vi "SendAndReceiveTest.vi"(8 "error in (no error)":errorcluster, 11 "SerialPortRef":T1) -> (0 "error out":errorcluster, 1 "Buffer":string, 3 "SerialPortRef 2":T1)   [LabVIEW 2015]
uses:
  <vilib>/Rock Robotics/WPI/SerialPort/WPI_SerialPortRef.ctl
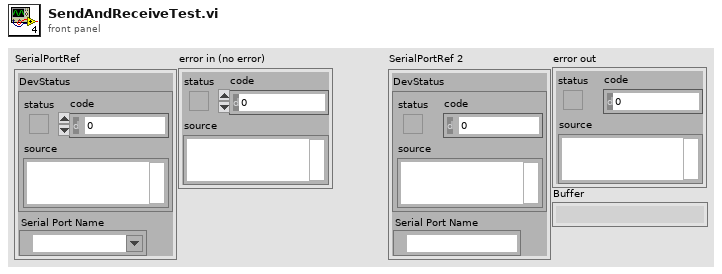
[diagram p1: front panel]
types:
  T1 = typedef "WPI_SerialPortRef.ctl" = cluster{"DevStatus":errorcluster, "Serial Port Name":refnum<visa-resource-name>}
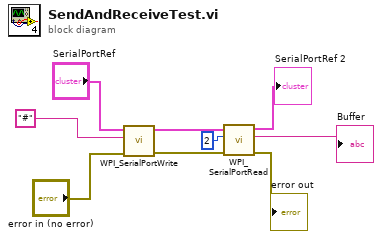
[diagram p0: block diagram]
diagram:
  n1 = call <vilib>:"WPI_SerialPortWrite.vi"("error in (no error)"="error in (no error)", "Buffer"="#", "SerialPortRef"="SerialPortRef") -> ("error out"=w8:errorcluster, "SerialPortRef"=w9:T1)  [unwired: 6 in, 1 out]
  n2 = call <vilib>:"WPI_SerialPortRead.vi"("error in (no error)"=w8, "Num Bytes to Read"=u32 2, "SerialPortRef"=w9) -> ("error out"=→"error out":errorcluster, "Buffer"=→"Buffer":string, "SerialPortRef"=→"SerialPortRef 2":T1)  [unwired: 6 in]
